vi "写入计数值.vi"(8 "error in (no error)":errorcluster, 9 "计数值":i32, 10 "通道":T1(ring), 11 "MB session in":refnum<class "MB_Master.lvclass">) -> (0 "error out":errorcluster, 3 "MB session out":refnum<class "MB_Master.lvclass">)   [LabVIEW 2016, in "DAM395CF.lvlib"]
uses:
  DAM395CF.lvlib
  <vilib>/Plasmionique/MB Master/MB_Master/MB_Master.lvclass
  <vilib>/Plasmionique/MB Master/MB Master.lvlib
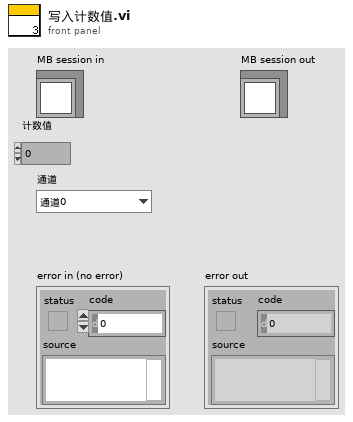
[diagram p1: front panel]
types:
  T1 = enum16{"通道0", "通道1", "通道2", "通道3", "通道4", "通道5", "通道6", "通道7"}
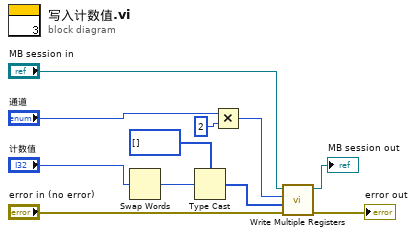
[diagram p0: block diagram]
diagram:
  n1 = Swap Words(1:"计数值") -> (0:w4:i32)
  n2 = Type Cast(type=u16[] [], x=w4) -> (*(type *) &x=w1:u16[])
  n3 = Multiply(x="通道", y=2) -> (x*y=w6:i32)
  n4 = call <vilib>:"Write Multiple Registers.vi"("error in (no error)"="error in (no error)", "values"=w1, "starting address"=w6, "MB session in"="MB session in") -> ("error out"=→"error out":errorcluster, "MB session out"=→"MB session out":refnum<class "MB_Master.lvclass">)  [unwired: 6 in]
